vi "_CallShell.vi"() -> ()   [LabVIEW 2019, in "lv-providershell-example3.lvlib"]
uses:
  lv-providershell-example3.lvlib
  Provider/ProviderClass.lvclass
  fd52217d-3635-4dc6-bc27-264ab1bf517b.vi
  fd52217d-3635-4dc6-bc27-264ab1bf517b.vi/dd404c74-838a-4847-8a35-f418c6f3a858.vi
  fd52217d-3635-4dc6-bc27-264ab1bf517b.vi/b72bd802-02c8-4c5c-a55b-cf878c87277d.vi
  fd52217d-3635-4dc6-bc27-264ab1bf517b.vi/265e1432-e678-43aa-bab0-a426ff8a1c8e.vi
  fd52217d-3635-4dc6-bc27-264ab1bf517b.vi/810081db-a115-4fe5-bf0e-384028abe08d.vi
  fd52217d-3635-4dc6-bc27-264ab1bf517b.vi/536915cd-a43e-403d-864d-25d72d4057e0.vi
  fd52217d-3635-4dc6-bc27-264ab1bf517b.vi/cd230284-44ce-4def-b757-1ac3d9066b09.vi
  src/_Support/__File Exists - Scalar__ogtk.vi
  src/_Support/__Strip Path Extension - String__ogtk.vi
  <vilib>/Utility/LVLibp/Get Exported File List.vi
  <vilib>/Utility/LVClass/Get LV Class Default Value.vi
  src/_Support/__Wait(ms) If Input Valid.vi
  <vilib>/Utility/libraryn.llb/Recursive File List.vi
  <vilib>/Utility/libraryn.llb/Check if File or Folder Exists.vi
  src/_Support/__Recursive File List with Exclude Option.vi
panel:
  out "Array 2":string[](array[string])
  out "Array":bool[](array[boolean])
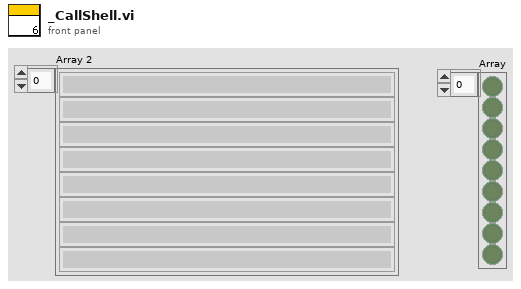
[diagram p1: front panel]
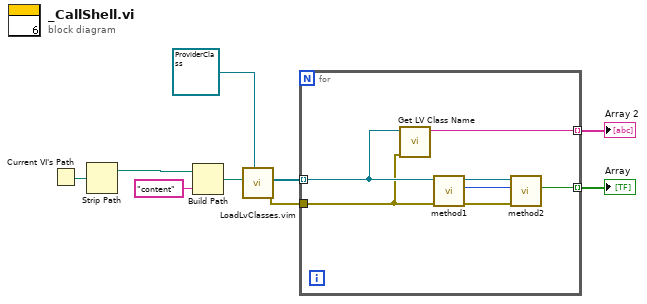
[diagram p0: block diagram]
diagram:
  n1 = Current VI's Path() -> (path=w2:path)
  n2 = Strip Path(path=w2) -> (stripped path=w1:path)  [unwired: 1 out]
  n3 = Build Path(base path=w1, name or relative path="content") -> (appended path=w7:path)
  n4 = call "LoadLvClasses.vim"("ClassType"=refnum<class "ProviderClass.lvclass"> refnum ("lv-providershell-example3.lvlib:ProviderClass.lvclass"), "Path"=w7) -> ("error out"=w4:errorcluster, "Loaded Classes"=w6:refnum<class "ProviderClass.lvclass">[])  [unwired: 8 in]
  n5 = for {
    tunnel: w6 -> [w12] mode=indexing
    tunnel: [w13] -> w5 mode=indexing
    tunnel: w4 -> [w11]
    tunnel: [w10] -> w3 mode=indexing
    n6 = call <vilib>:"Get LV Class Name.vi"("error in (no error)"=w11, "object"=w12) -> ("class name"=w10:string)  [unwired: 8 in, 1 out]
    n7 = call-dynamic "method1.vi"("error in (no error)"=w11, "ProviderClass in"=w12) -> ("error out"=w14:errorcluster, "RefNum"=w15:i32, "ProviderClass out"=w16:refnum<class "ProviderClass.lvclass">)  [unwired: 7 in]
    n8 = call-dynamic "method2.vi"("error in (no error)"=w14, "RefNum"=w15, "ProviderClass in"=w16) -> ("Boolean"=w13:bool)  [unwired: 6 in, 2 out]
  }
  "Array" <- w5
  "Array 2" <- w3
